vi "Calculate E.vi"(9 "Amplitude":dbl, 10 "amax":dbl) -> (2 "E":i32)   [LabVIEW 2014]
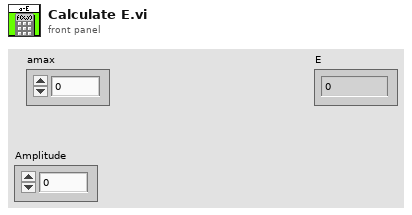
[diagram p1: front panel]
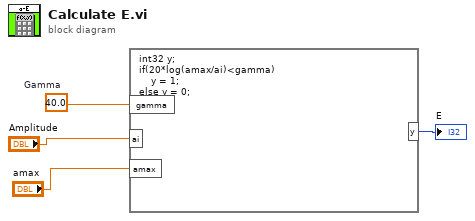
[diagram p0: block diagram]
diagram:
  w4 = 40.0  # Gamma
  n1 = formula code="int32 y;\nif(20*log(amax/ai)<gamma)\n    y = 1;\nelse y = 0;"("ai"="Amplitude", "amax"="amax", "gamma"=w4) -> ("y"=→"E":i32)
